vi "pendulo.vi"() -> ()   [LabVIEW 2013]
uses:
  <vilib>/Quanser/Rapid Control Prototyping Toolkit/hardware/HIL Board/_TypeSpecific/HIL Write Analog (Scalar).vi
  <vilib>/Quanser/Rapid Control Prototyping Toolkit/hardware/HIL Board/_TypeSpecific/HIL Read Encoder (Vector).vi
  <vilib>/Quanser/Rapid Control Prototyping Toolkit/hardware/HIL Board/HIL Board.lvclass
panel:
  out "t":dbl
  in  "Filtered/Raw":bool
  out "dbetaFIL":dbl
  out "dalphaFIL":dbl
  out "DefautCode":string="/*Para estabilizar arriba*/\nk1=-2.0;\nk2=35.0;\nk3=-1.5;\nk4=3.0;\n/*solo controlo ariba*/\nu[0]=-k1*(beta-consigna)-k2*alpha-k3*dbeta-k4*dalpha;\n\n/*para el swing up*/\nfunction sign(x) { return x > 0 ? 1 : x < 0 ? -1 : 1; }\nmu=50;//swing up gain\numax=6;\nEr=30.0/1000;\n\nMp=0.024;\nLp=0.127;\nJp=3.226e-5;\ng=9.81;\n\nMr=0.1;\nLr=0.095;\nR=6.3;\nkt=0.036;\n/*calculo la energía*/\nalpha2=alpha+Math.PI;\nEk = 0.5*Jp*dalpha*dalpha;\nEp = 0.5*Mp*g*Lp*(1-Math.cos(alpha2));\nE = Ek+Ep;\n/*y ahora el control*/\ntau=sign(Math.cos(alpha2)*dalpha)*mu*(E-Er);\n/*saturo*/\n//if (tau<-umax) tau=-umax;\n//if (tau>umax) tau=umax;\n/*por fin calculo u*/\nus=Mr*Lr*R*tau/kt\n\n//uso uno u otro dependiendo del ángulo (20 grados)\nif (Math.abs(alpha)>0.35) {u[0]=us;}\n//saco la energia para verla\nu[1]=E;\n"
  in  "Custom/Default":bool=TRUE
  in  "StudentCode":string
  out "Code":string="/*Para estabilizar arriba*/\nk1=-2.0;\nk2=35.0;\nk3=-1.5;\nk4=3.0;\n/*solo controlo ariba*/\nu[0]=-k1*(beta-consigna)-k2*alpha-k3*dbeta-k4*dalpha;\n\n/*para el swing up*/\nfunction sign(x) { return x > 0 ? 1 : x < 0 ? -1 : 1; }\nmu=50;//swing up gain\numax=6;\nEr=30.0/1000;\n\nMp=0.024;\nLp=0.127;\nJp=3.226e-5;\ng=9.81;\n\nMr=0.1;\nLr=0.095;\nR=6.3;\nkt=0.036;\n/*calculo la energía*/\nalpha2=alpha+Math.PI;\nEk = 0.5*Jp*dalpha*dalpha;\nEp = 0.5*Mp*g*Lp*(1-Math.cos(alpha2));\nE = Ek+Ep;\n/*y ahora el control*/\ntau=sign(Math.cos(alpha2)*dalpha)*mu*(E-Er);\n/*saturo*/\n//if (tau<-umax) tau=-umax;\n//if (tau>umax) tau=umax;\n/*por fin calculo u*/\nus=Mr*Lr*R*tau/kt\n\n//uso uno u otro dependiendo del ángulo (20 grados)\nif (Math.abs(alpha)>0.35) {u[0]=us;}\n//saco la energia para verla\nu[1]=E;\n"
  out "ControllerError":errorcluster
  out "PlantError":errorcluster
  out "Offest alpha":dbl=-1024.0
  out "Offest beta":dbl=-32.0
  out "Calibrating":bool
  in  "betaRef":dbl(slide) scale=-1.5..1.5
  out "t_ant":u32=1719669212
  out "alpha":dbl(graph)=-0.006135923151542565
  out "beta":dbl(graph)=-0.10431069357622362
  out "dalpha":dbl(graph)
  out "dbeta":dbl(graph)
  out "controlState":dbl[](array[numeric])=[0.006135904999999969, 0.029900598562205914]
  out "alphaANT":dbl=-0.006135923151542565
  out "betaANT":dbl=-0.10431069357622362
  out "u":dbl(graph)=0.006135904999999969
  in  "stop":bool
  in  "Period":i32=10
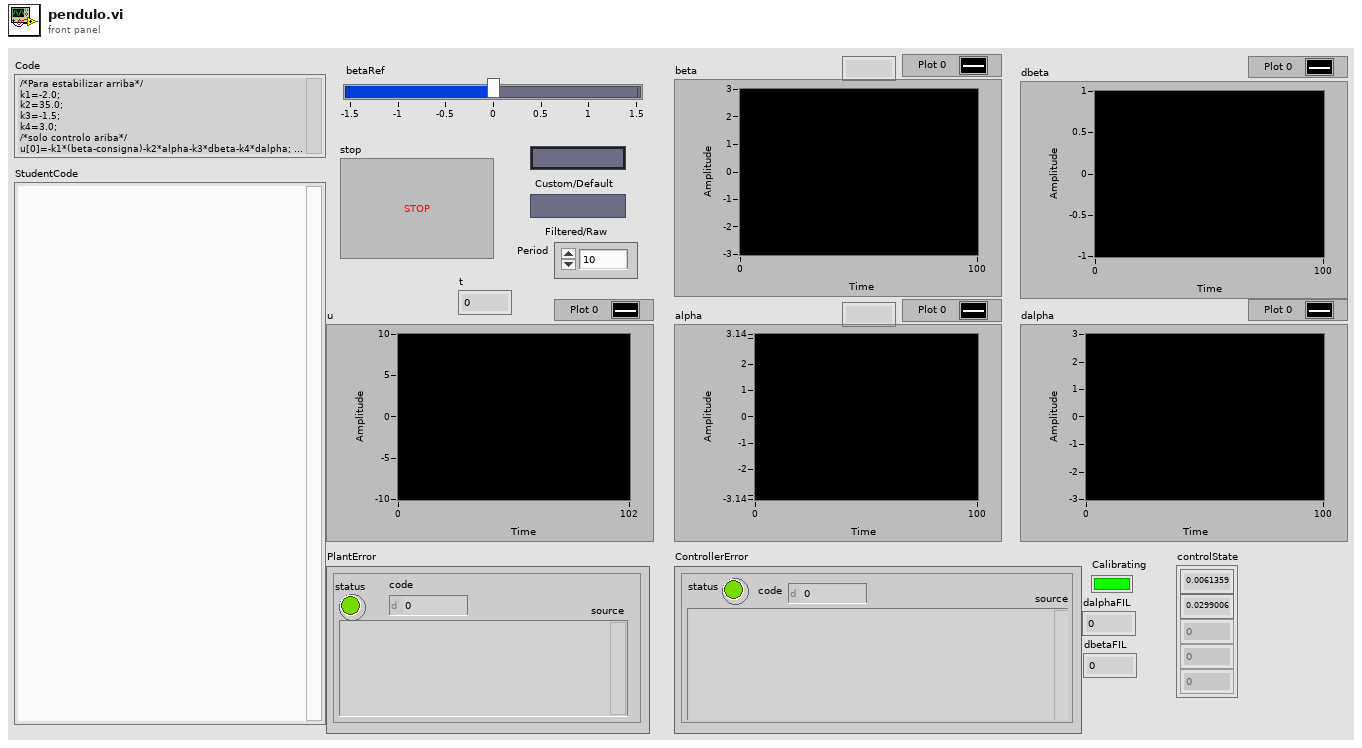
[diagram p1: front panel]
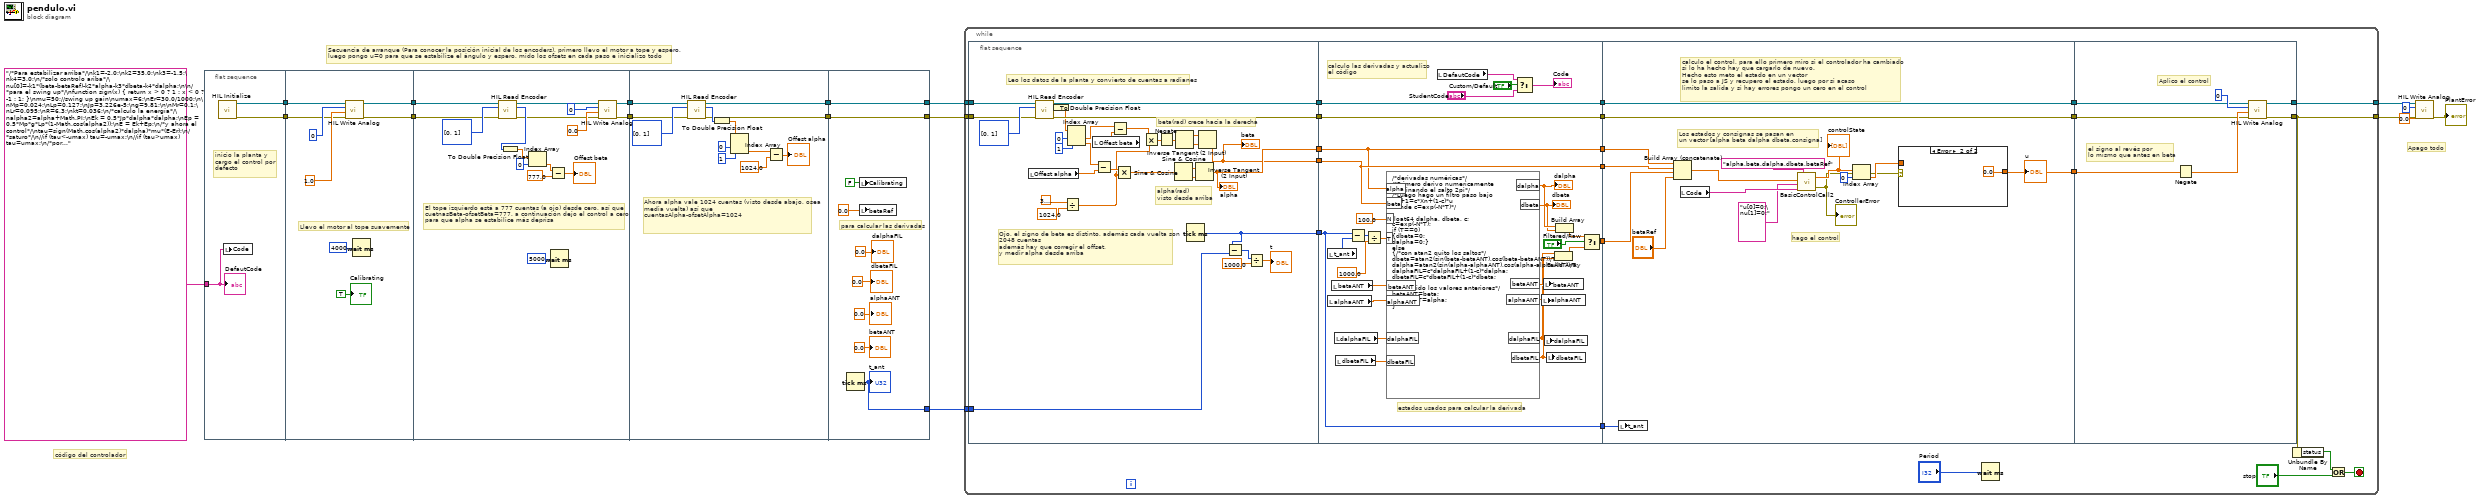
[diagram p0: block diagram]
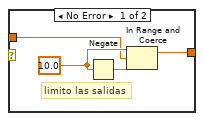
[diagram p2: hidden frame]
diagram:
  # "Secuencia de arranque (Para conocer la posición inicial de los encoders), primero llevo el motor a tope y espero, \nluego pongo u=0 para que se estabilize el ángulo y espero, mido los ofsets en cada paso e inicializo todo"
  # "código del controlador"
  # "Apago todo"
  n1 = flat-sequence {
    tunnel: [w20] -> w12
    tunnel: [w19] -> w11
    tunnel: "/*Para estabilizar arriba*/\nk1=-2.0;\nk2=35.0;\nk3=-1.5;\nk4=3.0;\n/*solo controlo ariba*/\nu[0]=-k1*(beta-betaRef)-k2*alpha-k3*dbeta-k4*dalpha;\n\n/*para el swing up*/\nfunction sign(x) { return x > 0 ? 1 : x < 0 ? -1 : 1; }\nmu=50;//swing up gain\numax=6;\nEr=30.0/1000;\n\nMp=0.024;\nLp=0.127;\nJp=3.226e-5;\ng=9.81;\n\nMr=0.1;\nLr=0.095;\nR=6.3;\nkt=0.036;\n/*calculo la energía*/\nalpha2=alpha+Math.PI;\nEk = 0.5*Jp*dalpha*dalpha;\nEp = 0.5*Mp*g*Lp*(1-Math.cos(alpha2));\nE = Ek+Ep;\n/*y ahora el control*/\ntau=sign(Math.cos(alpha2)*dalpha)*mu*(E-Er);\n/*saturo*/\n//if (tau<-umax) tau=-umax;\n//if (tau>umax) tau=umax;\n/*por fin calculo u*/\nus=Mr*Lr*R*tau/kt\n\n//uso uno u otro dependiendo del ángulo (20 grados)\nif (Math.abs(alpha)>0.35) {u[0]=us;}\n//saco la energia para verla\nu[1]=E;\n" ("Code") -> [w18]
    tunnel: w12 -> [w25]
    tunnel: [w22] -> w8
    tunnel: w11 -> [w24]
    tunnel: [w21] -> w7
    tunnel: w8 -> [w40]
    tunnel: w7 -> [w39]
    tunnel: [w30] -> w6
    tunnel: [w31] -> w5
    tunnel: [w46] -> w10
    tunnel: w6 -> [w53]
    tunnel: [w45] -> w9
    tunnel: w5 -> [w54]
    tunnel: w10 -> [w62]
    tunnel: w9 -> [w61]
    tunnel: [w62] -> w14
    tunnel: [w61] -> w13
    tunnel: [w57] -> w1
    frame #0 {
      # "inicio la planta y \ncargo el control por\ndefecto"
      n2 = call "HIL Initialize"() -> ("board out"=w20:refnum<class "HIL Board.lvclass">, "error out"=w19:errorcluster)  [unwired: 14 in]
      n3 = local write "Code"(w18) -> ()
      "DefautCode" <- w18
    }
    frame #1 {
      # "Llevo el motor al tope suavemente"
      n4 = call-poly <vilib>:"HIL Write Analog.vi"("error in (no error)"=w24, "voltage"=1.0, "channel"=u32 0, "board in"=w25) -> ("error out"=w21:errorcluster, "board out"=w22:refnum<class "HIL Board.lvclass">)  [unwired: 6 in]
      n5 = Wait (ms)(milliseconds to wait=u32 4000) -> ()  [unwired: 1 out]
      "Calibrating" <- TRUE ("Calibrando")
    }
    frame #2 {
      # "El tope izquierdo está a 777 cuentas (a ojo) desde cero, así que\ncuetnasBeta-ofsetBeta=777, a continuación dejo el control a cero\npara que alpha se estabilice más deprisa"
      n6 = call-poly <vilib>:"HIL Read Encoder.vi"("error in (no error)"=w39, "channels"=u32[] [0, 1], "board in"=w40) -> ("error out"=w32:errorcluster, "counts"=w41:i32[], "board out"=w33:refnum<class "HIL Board.lvclass">)  [unwired: 6 in]
      n7 = To Double Precision Float(number=w41) -> (double precision float=w38:dbl[])
      n8 = Index Array(array=w38, index=0) -> (element=w36:dbl)
      n9 = Subtract(x=w36, y=777.0) -> (x-y=→"Offest beta":dbl)
      n10 = Wait (ms)(milliseconds to wait=u32 5000) -> ()  [unwired: 1 out]
      n11 = call-poly <vilib>:"HIL Write Analog.vi"("error in (no error)"=w32, "voltage"=0.0, "channel"=u32 0, "board in"=w33) -> ("error out"=w30:errorcluster, "board out"=w31:refnum<class "HIL Board.lvclass">)  [unwired: 6 in]
    }
    frame #3 {
      # "Ahora alpha vale 1024 cuentas (visto desde abajo, osea\nmedia vuelta) así que \ncuentasAlpha-ofsetAlpha=1024"
      n12 = call-poly <vilib>:"HIL Read Encoder.vi"("error in (no error)"=w53, "channels"=u32[] [0, 1], "board in"=w54) -> ("error out"=w45:errorcluster, "counts"=w50:i32[], "board out"=w46:refnum<class "HIL Board.lvclass">)  [unwired: 6 in]
      n13 = To Double Precision Float(number=w50) -> (double precision float=w51:dbl[])
      n14 = Index Array(array=w51, index #1=0 ("index"), index #2=1 ("index")) -> (element #2=w48:dbl)  [unwired: 1 out]
      n15 = Subtract(x=w48, y=1024.0) -> (x-y=→"Offest alpha":dbl)
    }
    frame #4 {
      # "para calcular las derivadas"
      n16 = Tick Count (ms)() -> (millisecond timer value=w57:u32)
      "t_ant" <- w57
      n17 = local write "Calibrating"(FALSE ("Calibrando")) -> ()
      n18 = local write "betaRef"(0.0 ("Consigna")) -> ()
      "betaANT" <- 0.0 ("betaANT")
      "alphaANT" <- 0.0 ("alphaANT")
      "dalphaFIL" <- 0.0 ("alphaX")
      "dbetaFIL" <- 0.0 ("betaX")
    }
  }
  n19 = while {
    tunnel: w14 -> [w87]
    tunnel: w13 -> [w86]
    tunnel: [w73] -> w15
    tunnel: [w71] -> w4
    tunnel: w1 -> [w66]
    stop <- w68 stop-if-true
    n20 = flat-sequence {
      tunnel: w87 -> [w117]
      tunnel: w86 -> [w116]
      tunnel: [w115] -> w85
      tunnel: [w114] -> w84
      tunnel: [w95] -> w83
      tunnel: [w90] -> w82
      tunnel: [w94] -> w72
      tunnel: w66 -> [w89]
      tunnel: w85 -> [w148]
      tunnel: w84 -> [w147]
      tunnel: w83 -> [w141]
      tunnel: w82 -> [w136]
      tunnel: [w148] -> w81
      tunnel: [w147] -> w80
      tunnel: [w141] -> w79
      tunnel: [w142] -> w78
      tunnel: [w136] -> w77
      tunnel: w72 -> [w142]
      tunnel: [w123] -> w67
      tunnel: w81 -> [w162]
      tunnel: w80 -> [w164]
      tunnel: w79 -> [w159]
      tunnel: w78 -> [w158]
      tunnel: w77 -> [w163]
      tunnel: [w162] -> w76
      tunnel: [w164] -> w75
      tunnel: [w160] -> w74
      tunnel: w67 -> [w157]
      tunnel: w76 -> [w174]
      tunnel: w75 -> [w173]
      tunnel: w74 -> [w172]
      tunnel: [w171] -> w71
      tunnel: [w170] -> w73
      frame #0 {
        # "Ojo, el signo de beta es distinto, además cada vuelta son\n2048 cuentas \nademás hay que corregir el offset, \ny medir alpha desde arriba"
        # "alpha(rad) \nvisto desde arriba"
        # "beta(rad) crece hacia la derecha"
        # "Leo los datos de la planta y convierto de cuentas a radianes"
        n21 = local read "Offest alpha"() -> (w112:dbl)
        n22 = call-poly <vilib>:"HIL Read Encoder.vi"("error in (no error)"=w116, "channels"=u32[] [0, 1], "board in"=w117) -> ("error out"=w114:errorcluster, "counts"=w108:i32[], "board out"=w115:refnum<class "HIL Board.lvclass">)  [unwired: 6 in]
        n23 = To Double Precision Float(number=w108) -> (double precision float=w107:dbl[])
        n24 = Divide(x=3.141592653589793, y=1024.0) -> (x/y=w99:dbl)
        n25 = Index Array(array=w107, index #1=0 ("index"), index #2=1 ("index")) -> (element #1=w106:dbl, element #2=w105:dbl)
        n26 = local read "Offest beta"() -> (w113:dbl)
        n27 = Subtract(x=w105, y=w112) -> (x-y=w102:dbl)
        n28 = Subtract(x=w106, y=w113) -> (x-y=w111:dbl)
        n29 = Multiply(x=w102, y=w99) -> (x*y=w96:dbl)
        n30 = Multiply(x=w111, y=w99) -> (x*y=w97:dbl)
        n31 = Negate(x=w97) -> (-x=w98:dbl)
        n32 = Sine & Cosine(0:w96) -> (1:w110:dbl, 2:w109:dbl)
        n33 = Sine & Cosine(0:w98) -> (1:w104:dbl, 2:w103:dbl)
        n34 = Tick Count (ms)() -> (millisecond timer value=w90:u32)
        n35 = Inverse Tangent (2 Input)(1:w109, 2:w110) -> (0:w95:dbl)
        "alpha" <- w95
        n36 = Inverse Tangent (2 Input)(1:w103, 2:w104) -> (0:w94:dbl)
        "beta" <- w94
        n37 = Subtract(x=w90, y=w89) -> (x-y=w91:u32)
        n38 = Divide(x=w91, y=1000.0) -> (x/y=→"t":dbl)
      }
      frame #1 {
        # "estados usados para calcular la derivada"
        # "calculo las derivadas y actualizo\nel código"
        n39 = local read "t_ant"() -> (w146:u32)
        n40 = local read "alphaANT"() -> (w139:dbl)
        n41 = local read "betaANT"() -> (w140:dbl)
        n42 = local read "dalphaFIL"() -> (w131:dbl)
        n43 = local read "dbetaFIL"() -> (w130:dbl)
        n44 = Subtract(x=w136, y=w146) -> (x-y=w143:u32)
        n45 = Divide(x=w143, y=1000.0) -> (x/y=w145:dbl)
        n46 = formula code="/*derivadas numéricas*/\n/*Primero derivo numericamente\neliminando el salto 2pi*/\n/*Luego hago un filtro paso bajo\nXn+1=c*Xn+(1-c)*u  \ndonde c=exp(-N*T)*/\n\nfloat64 dalpha, dbeta, c;\nc=exp(-N*T);\nif (T==0)\n{dbeta=0;\ndalpha=0;}\nelse\n{/*con atan2 quito los saltos*/\ndbeta=atan2(sin(beta-betaANT),cos(beta-betaANT))/T;\ndalpha=atan2(sin(alpha-alphaANT),cos(alpha-alphaANT))/T;\ndalphaFIL=c*dalphaFIL+(1-c)*dalpha;\ndbetaFIL=c*dbetaFIL+(1-c)*dbeta;\n\n/*actualido los valores anteriores*/\nbetaANT=beta;\nalphaANT=alpha;\n}"("beta"=w142, "alpha"=w141, "T"=w145, "betaANT"=w140, "alphaANT"=w139, "N"=100.0 ("FilterConstant"), "dalphaFIL"=w131, "dbetaFIL"=w130) -> ("dbeta"=w128:dbl, "dalpha"=w129:dbl, "betaANT"=w137:dbl, "alphaANT"=w138:dbl, "dalphaFIL"=w126:dbl, "dbetaFIL"=w127:dbl)
        "dalpha" <- w129
        "dbeta" <- w128
        n47 = local read "DefautCode"() -> (w134:string)
        n48 = Select(t=w134, s="Custom/Default", f="StudentCode") -> (s? t:f=→"Code":string)
        n49 = local write "alphaANT"(w138) -> ()
        n50 = local write "betaANT"(w137) -> ()
        n51 = local write "dalphaFIL"(w126) -> ()
        n52 = local write "dbetaFIL"(w127) -> ()
        n53 = Build Array(w126, w127) -> (w124:dbl[])
        n54 = Build Array(w129, w128) -> (w125:dbl[])
        n55 = Select(t=w125, s="Filtered/Raw", f=w124) -> (s? t:f=w123:dbl[])
      }
      frame #2 {
        # "hago el control"
        # "Los estados y consignas se pasan en \nun vector [alpha beta dalpha dbeta,consigna]"
        # "calculo el control, para ello primero miro si el controlador ha cambiado\nsi lo ha hecho hay que cargarlo de nuevo.\nHecho esto meto el estado en un vector\nse lo paso a JS y recupero el estado, luego por si acaso \nlimito la salida y si hay errores pongo un cero en el control"
        n56 = local write "t_ant"(w163) -> ()
        n57 = Build Array (concatenate)(w159, w158, w157, "betaRef") -> (w153:dbl[])
        n58 = local read "Code"() -> (w154:string)
        n59 = call "BasicControlCall2.vi"("Code"=w154, "InitCode"="u[0]=0;\nu[1]=0;", "plantState"=w153, "variablesIN"="alpha,beta,dalpha,dbeta,betaRef") -> ("error"=w149:errorcluster, "controlState"=w150:dbl[])
        "controlState" <- w150
        "ControllerError" <- w149
        n60 = Index Array(array=w150, index=0) -> (element=w161:dbl)
        n61 = case shown="Error" w149 {
          tunnel: w161 -> [w165 _]
          tunnel: [w166 0.0 ("default (0 dbl)")] -> w160
          frame No Error {
            w167 = 10.0 ("x")
            # "limito las salidas"
            n62 = Negate(x=w167) -> (-x=w168:dbl)
            n63 = In Range and Coerce(upper limit=w167, x=w165, lower limit=w168) -> (coerced(x)=w166:dbl)  [unwired: 1 out]
          }
          frame Error {
          }
        }
        "u" <- w160
      }
      frame #3 {
        # "el signo al revés por \nlo mismo que antes en beta"
        # "Aplico el control"
        n64 = Negate(x=w172) -> (-x=w176:dbl)
        n65 = call-poly <vilib>:"HIL Write Analog.vi"("error in (no error)"=w173, "voltage"=w176, "channel"=u32 0, "board in"=w174) -> ("error out"=w171:errorcluster, "board out"=w170:refnum<class "HIL Board.lvclass">)  [unwired: 6 in]
      }
    }
    n66 = Wait (ms)(milliseconds to wait="Period") -> ()  [unwired: 1 out]
    n67 = Unbundle By Name(w71) -> ("status"=w69:bool)
    n68 = Or(x=w69, y="stop") -> (x .or. y?=w68:bool)
  }
  n69 = call-poly <vilib>:"HIL Write Analog.vi"("error in (no error)"=w4, "voltage"=0.0, "channel"=u32 0, "board in"=w15) -> ("error out"=→"PlantError":errorcluster)  [unwired: 6 in, 1 out]
